vi "내컴퓨터.vi"() -> ()   [LabVIEW 2014]
panel:
  out "추가된 배열":string[](array[string])=["Windows NT", "6.1", "7601", "Windows 7 Professional Service Pack 1", "Samsung SCX-3200 Series"]
  in  "머신이름":string="192.168.0.79"
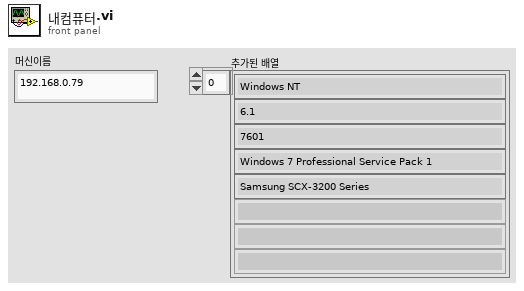
[diagram p1: front panel]
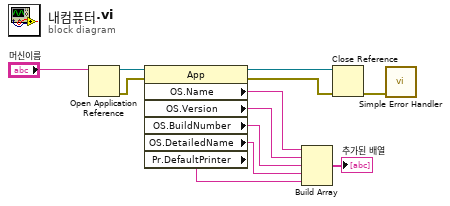
[diagram p0: block diagram]
diagram:
  n1 = Open Application Reference(11:"머신이름") -> (0:w10:errorcluster, 3:w12:refnum<vi>)  [unwired: 3 in]
  n2 = property class="App"(reference=w12, error in=w10) -> (reference out=w11:refnum<vi>, error out=w9:errorcluster, "OS.Name"=w7:string, "OS.Version"=w6:string, "OS.BuildNumber"=w5:string, "OS.DetailedName"=w4:string, "Pr.DefaultPrinter"=w3:string)
  n3 = Build Array(w7, w6, w5, w4, w3) -> (→"추가된 배열":string[])
  n4 = Close Reference(reference=w11, error in (no error)=w9) -> (error out=w8:errorcluster)
  n5 = call <vilib>:"Simple Error Handler.vi"("error in (no error)"=w8) -> ()  [unwired: 4 in, 5 out]
